vi "ZGenerate.vi"() -> ()   [LabVIEW 2016]
uses:
  <vilib>/Analysis/NI_AALPro.lvlib
  <vilib>/Analysis/polynomials.llb/Unique Numbers and Multiplicity (DBL).vi
panel:
  in  "Manual '# fields'":i32=1
  in  "Tab Control":enum32{"Page 1", "Page 2"}(tab)
  in  "IV file name distinction":string="decimated_21-BG+SG_Sweep+OVERNIGHT"
  in  "Processed data folder":path=path "B:/SketchSET/SA03008H.20180718/processed"
  in  "# of fields/Temperatures":i32=1
  in  "Field Period":i32=1
  in  "File or Folder Path":path=path "D:/SA03008H.20180718/58-SG_-1to1_0.025steps_@4T_at.2Hz_-300mVto100mV_IV"
  in  "Additional comments":string
  in  "IV setup":T1={"# of Vslow"=101, "# Vfast"=41, "#IV Curves at each gate"=1, "B/T offset"=0, "Discard first # curves"=0, "Manual offset"=0}
  in  "Scan names":string[](array[string])=["DSA_Vsg1", "B", "B"]
  in  "Portion of data":cluster{dbl, dbl}(slide)={1.0, 0.0} scale=0.0..1.0
  in  "Decimate point":dbl=10.0 format="%#_1f"
  in  "T/B     third axis":bool
  in  "Extract parameters from comments?":bool=TRUE
  in  "index 2":T2={"A"=3, "B"=5, "C"=3, "D"=5, "E"=3, "N1"=2, "N2"=2, "N3"=3, "N4"=4, "A 1"=3, "A 2"=3, "C 1"=3, "C 2"=3, "E 2"=4}
  # "This gets added to the original data name, then a number for individuality"
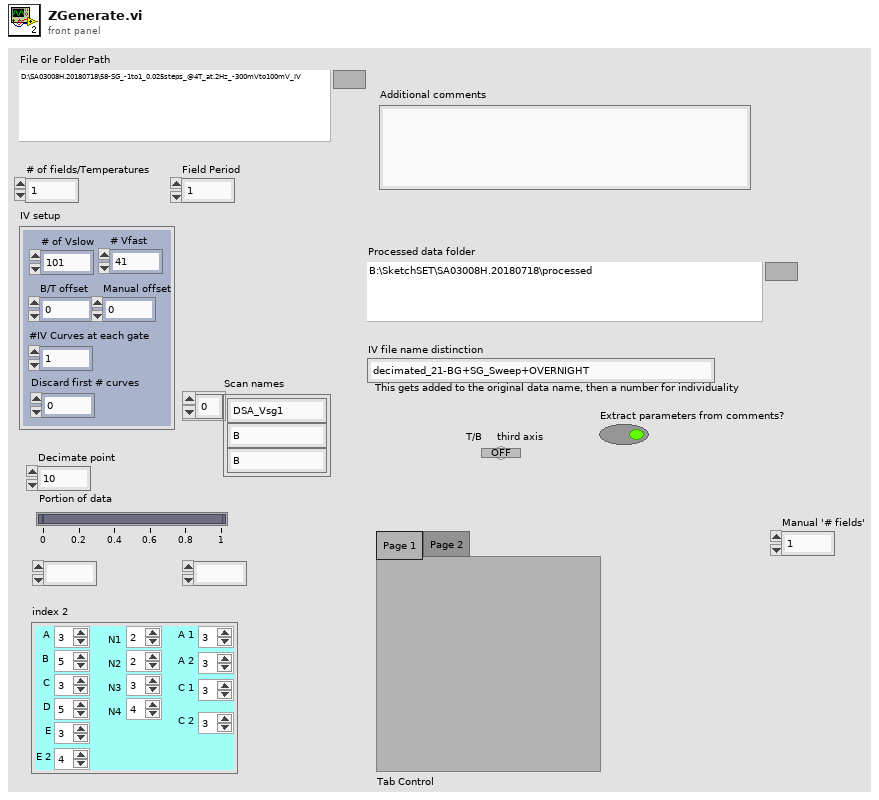
[diagram p1: front panel]
types:
  T1 = cluster{"# of Vslow":i32, "# Vfast":i32, "#IV Curves at each gate":i32, "B/T offset":i32, "Discard first # curves":i32, "Manual offset":i32}
  T2 = cluster{"A":i32, "B":i32, "C":i32, "D":i32, "E":i32, "N1":i32, "N2":i32, "N3":i32, "N4":i32, "A 1":i32, "A 2":i32, "C 1":i32, "C 2":i32, "E 2":i32}
  T3 = enum16{"open", "replace", "create", "open or create", "replace or create", "replace or create with confirmation"}
  T4 = typedef "SweepControl.lvclass/ScanControl.ctl" = T5[]
  T5 = typedef "SweepControl.lvclass/Cluster - ScanControl.ctl" = cluster{"Priority":T6, "Scan name":T7}
  T6 = typedef "SweepControl.lvclass/Enum - Priority.ctl" = enum16{"Priority 0", "Priority 1", "Priority 2", "Priority 3", "Priority 4", "Priority 5"}
  T7 = typedef "SweepControl.lvclass/Enum - Action.ctl" = enum16{"OFF", "DSA_Vamp", "DSA_freq", "DSA_Vsg1", "DSA_Vsg2", "DSA_Vsg3", "DAQ_Vbg", "B_Field", "Humidity", "Temp", "MW_freq1", "MW_freq2", "MW_amplitude1", "MW_amplitude2"}
  T8 = typedef "SweepControl.lvclass/ScanParamters.ctl" = T9[]
  T9 = typedef "SweepControl.lvclass/Cluster - ScanParamters.ctl" = cluster{"Start":dbl, "End":dbl, "Step":dbl, "Rate":dbl, "wait (ms)":u32, "address":refnum<visa-resource-name>, "Channel":i32}
  T10 = cluster{"Sorted scan control":cluster{T4}[], "Sorted scan parameters":cluster{T8}[], "# Of Sweep Pts. Fast to Slow":i16[]}
  T11 = cluster{"IV":cluster{dbl[], dbl[]}[][][], "IV-2T":cluster{dbl[], dbl[]}[][][], "Vfast":dbl[][], "Vslow":dbl[], dbl[], string, "Scan names":string[]}
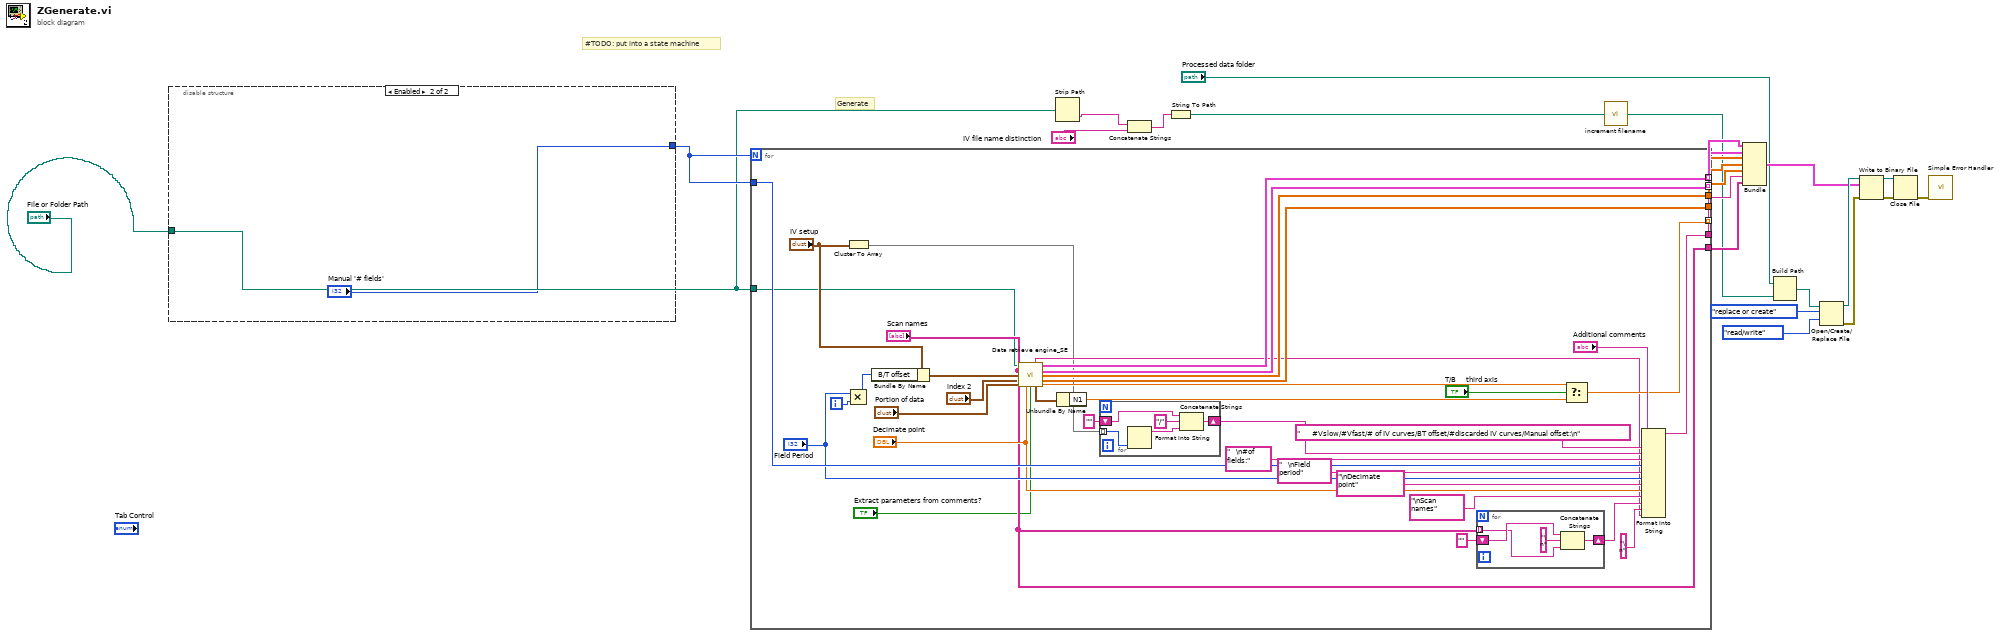
[diagram p0: block diagram]
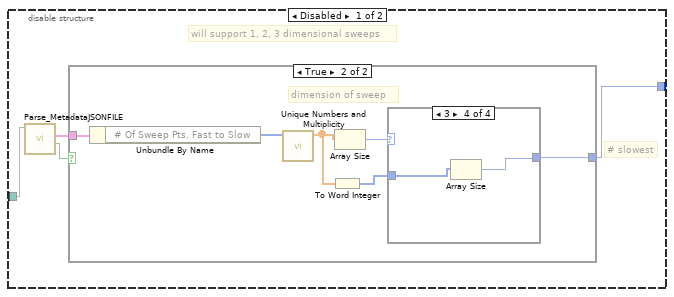
[diagram p2: hidden frame]
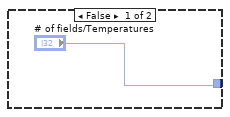
[diagram p3: hidden frame]
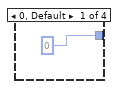
[diagram p4: hidden frame]
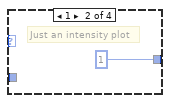
[diagram p5: hidden frame]
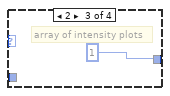
[diagram p6: hidden frame]
diagram:
  # "#TODO: put into a state machine"
  # "Generate"
  n1 = disable-structure shown="Enabled" {
    disable-tunnel: [w27 "Manual '# fields'"] -> w7
    disable-tunnel: "File or Folder Path" -> [w25 _]
    frame Disabled {
      # "will support 1, 2, 3 dimensional sweeps"
      # "# slowest"
      n2 = call "Parse_MetadataJSONFILE.vi"("File or Folder Path"=w25) -> ("file or folder exists?"=w26:bool, "output cluster"=w28:T10)  [unwired: 8 in, 1 out]
      n3 = case shown="True" w26 {
        tunnel: w28 -> [_ w35]
        tunnel: ["# of fields/Temperatures" w32] -> w27
        frame False {
        }
        frame True {
          # "dimension of sweep"
          n4 = Unbundle By Name(w35) -> ("# Of Sweep Pts. Fast to Slow"=w34:i16[])
          n5 = call-poly <vilib>:"Unique Numbers and Multiplicity.vi"("Numbers"=w34) -> ("Unique Numbers"=w31:dbl[])  [unwired: 8 in, 2 out]
          n6 = To Word Integer(number=w31) -> (16bit integer=w30:i16[])
          n7 = Array Size(array=w31) -> (size(s)=w33:i32)
          n8 = case shown="3" w33 {
            tunnel: [0 1 1 w40] -> w32
            tunnel: w30 -> [_ _ _ w39]
            frame 0, Default {
            }
            frame 1 {
              # "Just an intensity plot"
            }
            frame 2 {
              # "array of intensity plots"
            }
            frame 3 {
              n9 = Array Size(array=w39) -> (size(s)=w40:i32)
            }
          }
        }
      }
    }
    frame Enabled {
    }
  }
  n10 = for {
    N: w7 -> [_]
    tunnel: [w76] -> w24 mode=indexing
    tunnel: [w72] -> w12
    tunnel: [w71] -> w11
    tunnel: [w70] -> w14 mode=indexing
    tunnel: [w53] -> w10 mode=indexing
    tunnel: w7 -> [w61]
    tunnel: [w52] -> w13
    tunnel: ["Scan names"] -> w9
    tunnel: "File or Folder Path" -> [w43]
    i -> [w75]
    n11 = Multiply(x="Field Period", y=w75) -> (x*y=w73:i32)
    n12 = Cluster To Array(cluster="IV setup") -> (array=w42:i32[])
    n13 = Bundle By Name(cluster="IV setup", "B/T offset"=w73) -> (w66:T1)
    n14 = call "Data retrieve engine_SE.vi"("File or Folder Path"=w43, "Scan names"="Scan names", "IV setup"=w66, "index"="index 2", "Portion of data"="Portion of data", "Decimate point"="Decimate point", "Extract paramaters from comments?"="Extract parameters from comments?") -> ("Comments"=w47:string, "IV"=w76:cluster{dbl[], dbl[]}[][], "IV-2T"=w70:cluster{dbl[], dbl[]}[][], "Vfast"=w72:dbl[][], "Vslow"=w71:dbl[], "N"=w74:cluster{"N1":dbl, "N2":dbl, "N3":dbl, "N4":dbl}, "Vslowest"=w56:dbl)  [unwired: 2 in]
    n15 = Unbundle By Name(w74) -> ("N1"=w55:dbl)
    n16 = for {
      tunnel: w42 -> [w85] mode=indexing
      shift-right: [w82] -> w63
      shift-left: "" -> [w81]
      n17 = Format Into String(w85) -> (resulting string=w84:string)  [unwired: 3 in, 1 out]
      n18 = Concatenate Strings(w81, "/" ("string"), w84) -> (w82:string)
    }
    n19 = for {
      tunnel: "Scan names" -> [w78] mode=indexing
      shift-right: [w80] -> w49
      shift-left: "" -> [w79]
      n20 = Concatenate Strings(w79, "\n" ("string"), w78) -> (w80:string)
    }
    n21 = Select(t=w56, s="T/B     third axis", f=w55) -> (s? t:f=w53:dbl)
    n22 = Format Into String(initial string="Additional comments", "      #Vslow/#Vfast/# of IV curves/BT offset/#discarded IV curves/Manual offset:\n" ("string"), w63, "   \n#of fields:" ("string"), w61, "   \nField period" ("string"), "Field Period", "\nDecimate point", "Decimate point", "\nScan names", w49, "\n" ("input 11"), w47) -> (resulting string=w52:string)  [unwired: 2 in, 1 out]
  }
  n23 = Strip Path(path="File or Folder Path") -> (name=w3:string)  [unwired: 1 out]
  n24 = Concatenate Strings(w3, "IV file name distinction") -> (w2:string)
  n25 = String To Path(string=w2) -> (path=w5:path)
  n26 = call <userlib>:"increment filename.vi"("path"=w5) -> ("modified path"=w1:path)
  n27 = Bundle("IV"=w24, "IV-2T"=w14, "Vfast"=w12, "Vslow"=w11, w10, w13, "Scan names"=w9) -> (w15:T11)  [unwired: 1 in]
  n28 = Build Path(base path="Processed data folder", name or relative path=w1) -> (appended path=w16:path)
  n29 = Open/Create/Replace File(file path (use dialog)=w16, operation (0:open)=T3."replace or create", access (0:read/write)=enum16{"read/write", "read-only", "write-only"}."read/write") -> (refnum out=w19:refnum<file>, error out=w20:errorcluster)  [unwired: 3 in, 1 out]
  n30 = Write to Binary File(file (use dialog)=w19, data=w15, error in=w20) -> (refnum out=w23:refnum<file>, error out=w22:errorcluster)  [unwired: 3 in, 1 out]
  n31 = Close File(refnum=w23, error in=w22) -> (error out=w21:errorcluster)  [unwired: 1 out]
  n32 = call <vilib>:"Simple Error Handler.vi"("error in (no error)"=w21) -> ()  [unwired: 4 in, 5 out]
